vi "Lidar Global.vi"() -> ()   [LabVIEW 2016]
panel:
  in  "Lidar Distance":u16
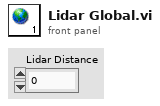
[diagram p1: front panel]
diagram:
